vi "ButtonCloseArms.vi"(11 "Buttons":bool[](array[boolean])) -> ()   [LabVIEW 2014]
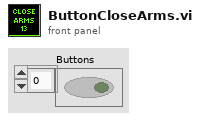
[diagram p1: front panel]
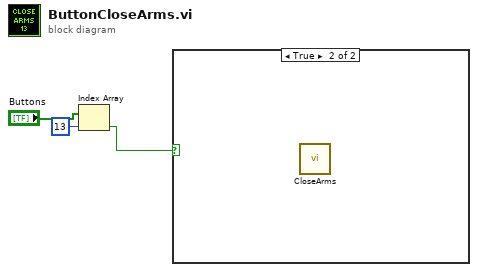
[diagram p0: block diagram]
diagram:
  n1 = Index Array(array="Buttons", index=13) -> (element=w1:bool)
  n2 = case shown="True" w1 {
    frame False {
    }
    frame True {
      n3 = call "CloseArms.vi"() -> ()  [unwired: 12 in]
    }
  }
